vi "CreateASCIIQueue.vi"() -> (3 "Queue out":refnum<queue>)   [LabVIEW 2013]
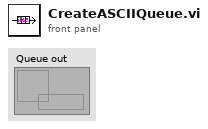
[diagram p1: front panel]
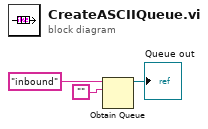
[diagram p0: block diagram]
diagram:
  n1 = Obtain Queue(name (unnamed)="inbound", element data type="") -> (queue out=→"Queue out":refnum<queue>)  [unwired: 3 in, 2 out]
